vi "Test Simple Server.vi"() -> ()   [LabVIEW 2020]
uses:
  HTTP Server/Server/Server.lvclass
  Test Index/Test Index.lvclass
  C:/dev/IlluminatedG/lv-http-server/HTTP Server/Handler/Handler.lvclass
panel:
  out "error out":errorcluster
  in  "Port":u16=36987
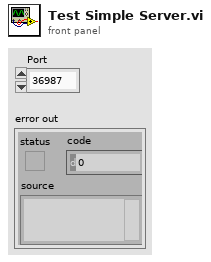
[diagram p1: front panel]
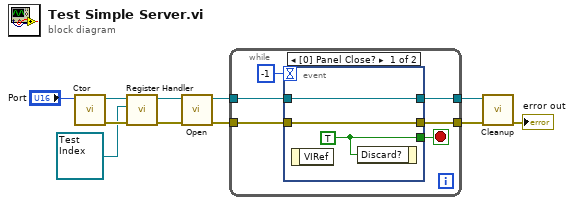
[diagram p0: block diagram]
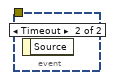
[diagram p2: hidden frame]
diagram:
  n1 = call "Ctor.vi"("Port (8080)"="Port") -> ("error out"=w2:errorcluster, "Server out"=w5:refnum<class "Server.lvclass">)  [unwired: 9 in]
  n2 = call "Register Handler.vi"("error in (no error)"=w2, "Handler"=refnum<class "Test Index.lvclass"> refnum ("Test Index.lvclass"), "Server in"=w5) -> ("error out"=w3:errorcluster, "Server out"=w4:refnum<class "Server.lvclass">)  [unwired: 7 in]
  n3 = call "Open.vi"("error in (no error)"=w3, "Server in"=w4) -> ("error out"=w9:errorcluster, "Server out"=w10:refnum<class "Server.lvclass">)  [unwired: 8 in]
  n4 = while {
    tunnel: w10 -> [w15]
    tunnel: w9 -> [w16]
    tunnel: [w14] -> w8
    tunnel: [w13] -> w7
    stop <- w17 stop-if-true
    n5 = event shown="[0] Panel Close?" {
      selector: _ -> [_ _]
      dyn-events: _ -> [_ _]
      timeout: -1 -> [_ _]
      tunnel: [w20 _] -> w17
      tunnel: w16 -> [w18 _]
      tunnel: w15 -> [w19 _]
      tunnel: [w19 _] -> w14
      tunnel: [w18 _] -> w13
      event Panel Close? {
        w20 = TRUE ("Discard?")
        n6 = event-data() -> ()  [unwired: 1 in, 1 out]
        n7 = event-data("Discard?"=w20) -> ()  [unwired: 1 in, 1 out]
      }
      event Timeout {
        n8 = event-data() -> ()  [unwired: 1 in, 1 out]
      }
    }
  }
  n9 = call "Cleanup.vi"("error in (no error)"=w7, "Server in"=w8) -> ("error out"=→"error out":errorcluster)  [unwired: 9 in]
